vi "set Thrust.vi"(9 "Held":bool, 10 "Thrust":bool, 11 "Control State in":refnum<class "Control State.lvclass">) -> (3 "Control State out":refnum<class "Control State.lvclass">)   [LabVIEW 2021, in "Control State.lvclass"]
uses:
  Control State.lvclass
  Control State.lvclass/Control State.ctl
  Button State.ctl
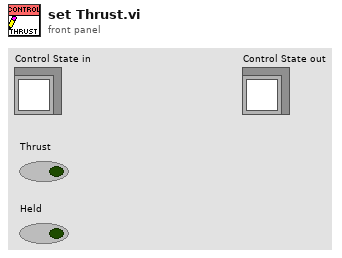
[diagram p1: front panel]
types:
  T1 = typedef "Control State.lvclass/Button State.ctl" = enum16{"Undefined", "Pressed", "Released", "Held", "Not Held"}
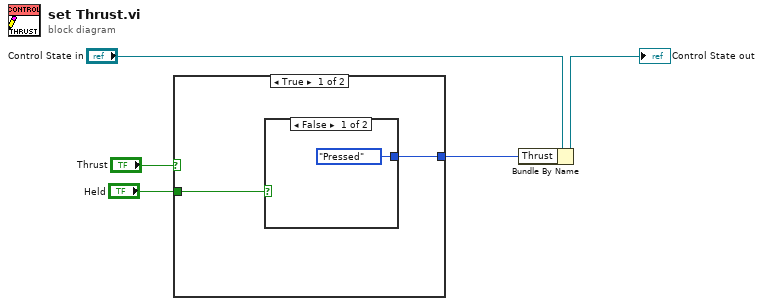
[diagram p0: block diagram]
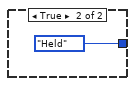
[diagram p2: hidden frame]
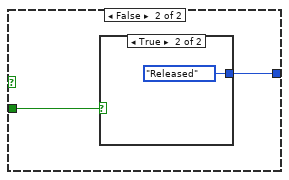
[diagram p3: hidden frame]
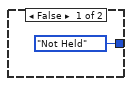
[diagram p4: hidden frame]
diagram:
  n1 = case shown="True" "Thrust" {
    tunnel: [w7 w11] -> w3
    tunnel: "Held" -> [w6 w10]
    frame True {
      n2 = case shown="False" w6 {
        tunnel: [Button_State."Pressed" ("Thrust") Button_State."Held" ("Thrust")] -> w7
        frame False {
        }
        frame True {
        }
      }
    }
    frame False {
      n3 = case shown="True" w10 {
        tunnel: [Button_State."Not Held" ("Thrust") Button_State."Released" ("Thrust")] -> w11
        frame False {
        }
        frame True {
        }
      }
    }
  }
  n4 = Bundle By Name(cluster="Control State in", "Thrust"=w3) -> (→"Control State out":refnum<class "Control State.lvclass">)
